vi "fgt get sensor Channel Count.vi"(8 "error in (no error)":errorcluster) -> (0 "error out":errorcluster, 3 "nbSChan out":u32)   [LabVIEW 2020, in "fgt_SDK.lvlib"]
doc: "Get total number of initialized sensor channels.\nIt is the sum of all connected flow-units on Flowboard, FlowEZ and IPS sensors"
uses:
  fgt_SDK.lvlib
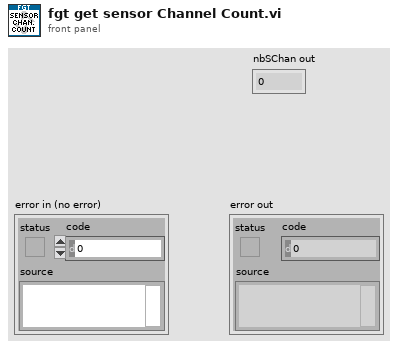
[diagram p1: front panel]
types:
  T1 = typedef "fgt_SDK.lvlib/fgt_STATUS_INFO.ctl" = cluster{"InstrType":T2, "instrSN":u16, "errorCode":u8, "infoCode":u8, "detail":string}
  T2 = typedef "fgt_SDK.lvlib/fgt_INSTRUMENT_TYPE.ctl" = enum32{"None", "MFCS", "MFCS_EZ", "FRP", "LineUP", "IPS"}
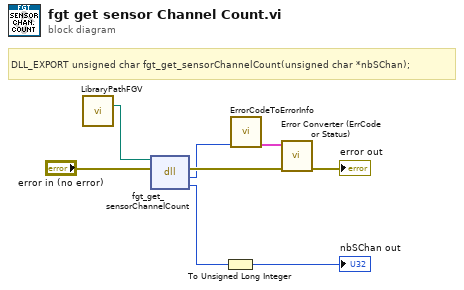
[diagram p0: block diagram]
diagram:
  # "DLL_EXPORT unsigned char fgt_get_sensorChannelCount(unsigned char *nbSChan);"
  n1 = call "LibraryPathFGV.vi"() -> ("Path Out"=w1:path)  [unwired: 14 in, 1 out]
  n2 = dll-call lib="C:/Workspace/fgt-SDK/LabVIEW/dlls/fgt_SDK_*.*" fn="fgt_get_sensorChannelCount"(path in=w1, error in="error in (no error)") -> (error out=w7:errorcluster, "return type"=w5:u8, "nbSChan"=w3:u8)  [unwired: 2 in, 1 out]
  n3 = To Unsigned Long Integer(number=w3) -> (unsigned 32bit integer=→"nbSChan out":u32)
  n4 = call "ErrorCodeToErrorInfo.vi"("return type"=w5) -> ("StatusInfo"=w4:T1)  [unwired: 10 in]
  n5 = call "Error Converter (ErrCode or Status).vi"("error in (no error)"=w7, "StatusInfo"=w4) -> ("error out"=→"error out":errorcluster)  [unwired: 9 in]
